vi "Set_All_Outputs.vi"(2 "error in":errorcluster, 3 "register 2 (8-13)":T1=[FALSE, FALSE, FALSE, FALSE, FALSE, FALSE], 4 "register 1 (2-7)":T2, 5 "VISA arduino in":refnum<visa-resource-name>) -> (0 "error out":errorcluster, 1 "VISA arduino out":refnum<visa-resource-name>)   [LabVIEW 2021]
uses:
  Register_1.ctl
  Register_2.ctl
  Delay_Global.vi
  <vilib>/Utility/error.llb/Error Cluster From Error Code.vi
  <vilib>/ErrorRing/Error Ring.xnode
panel:
  out "delay":u32
  out "comand 2":string
  out "comand 1":string
  # "Private"
  # "Public"
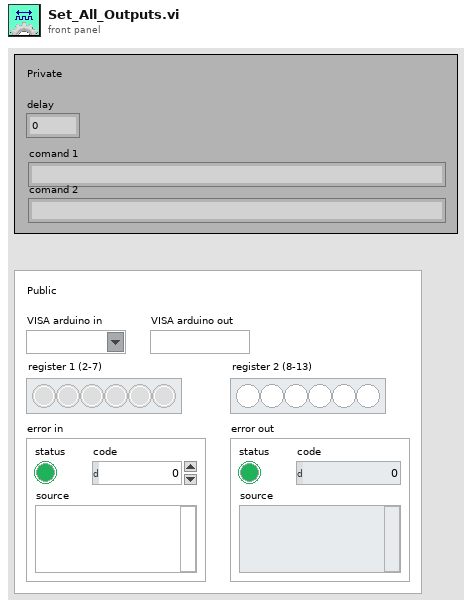
[diagram p1: front panel]
types:
  T1 = typedef "Register_2.ctl" = bool[]
  T2 = typedef "Register_1.ctl" = bool[]
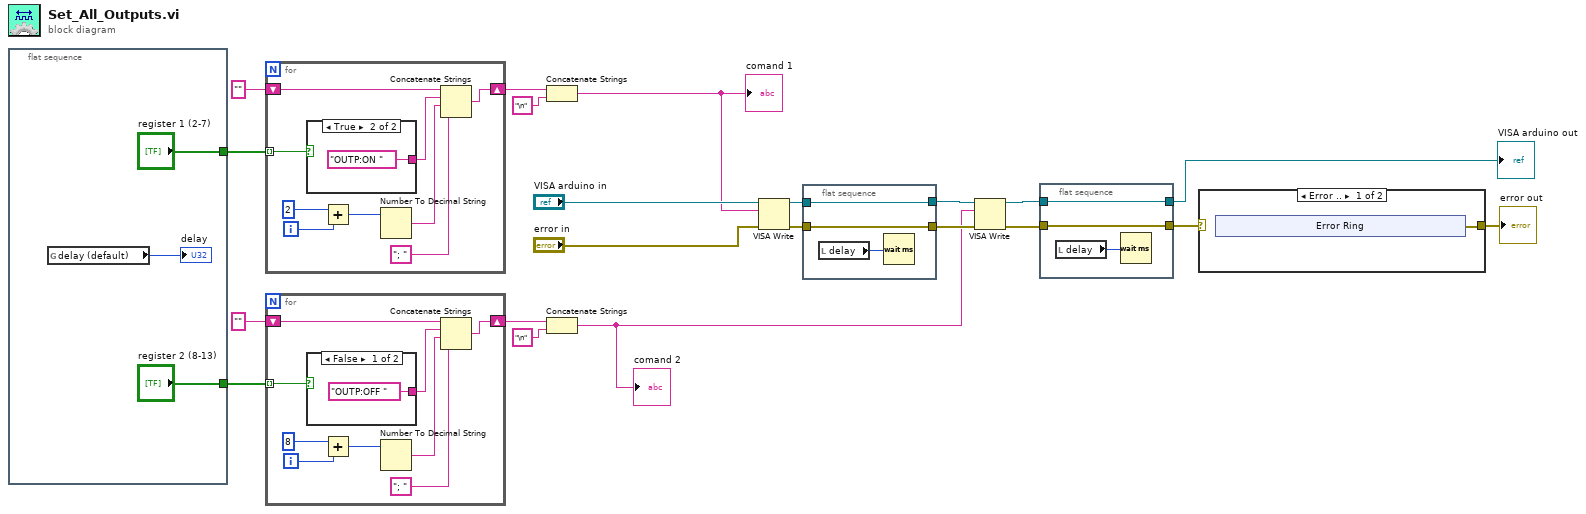
[diagram p0: block diagram]
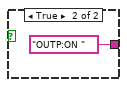
[diagram p3: hidden frame]
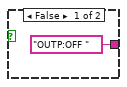
[diagram p4: hidden frame]
diagram:
  n1 = flat-sequence {
    tunnel: ["register 1 (2-7)"] -> w21
    tunnel: ["register 2 (8-13)"] -> w14
    frame #0 {
      n2 = global read "Delay_Global.vi" "delay (default)"() -> (→"delay":u32)
    }
  }
  n3 = for {
    shift-right: [w29] -> w18
    shift-left: "" -> [w28]
    tunnel: w21 -> [w33] mode=indexing
    i -> [w31]
    n4 = case shown="True" w33 {
      tunnel: ["OUTP:OFF " "OUTP:ON "] -> w27
      frame False {
      }
      frame True {
      }
    }
    n5 = Add(x=2, y=w31) -> (x+y=w30:i32)
    n6 = Number To Decimal String(number=w30) -> (decimal integer string=w26:string)  [unwired: 1 in]
    n7 = Concatenate Strings(w28, w27, w26, "; ") -> (w29:string)
  }
  n8 = for {
    shift-right: [w40] -> w17
    shift-left: "" -> [w39]
    tunnel: w14 -> [w44] mode=indexing
    i -> [w42]
    n9 = case shown="False" w44 {
      tunnel: ["OUTP:OFF " "OUTP:ON "] -> w38
      frame False {
      }
      frame True {
      }
    }
    n10 = Add(x=8, y=w42) -> (x+y=w41:i32)
    n11 = Number To Decimal String(number=w41) -> (decimal integer string=w37:string)  [unwired: 1 in]
    n12 = Concatenate Strings(w39, w38, w37, "; ") -> (w40:string)
  }
  n13 = Concatenate Strings(w18, "\n" ("string")) -> (w11:string)
  "comand 1" <- w11
  n14 = Concatenate Strings(w17, "\n" ("string")) -> (w6:string)
  "comand 2" <- w6
  n15 = VISA Write(VISA resource name="VISA arduino in", write buffer=w11, error in (no error)="error in") -> (VISA resource name out=w10:refnum<visa-resource-name>, error out=w9:errorcluster)  [unwired: 1 out]
  n16 = flat-sequence {
    tunnel: w10 -> [w48]
    tunnel: w9 -> [w47]
    tunnel: [w48] -> w8
    tunnel: [w47] -> w7
    frame #0 {
      n17 = local read "delay"() -> (w49:u32)
      n18 = Wait (ms)(milliseconds to wait=w49) -> ()  [unwired: 1 out]
    }
  }
  n19 = VISA Write(VISA resource name=w8, write buffer=w6, error in (no error)=w7) -> (VISA resource name out=w5:refnum<visa-resource-name>, error out=w4:errorcluster)  [unwired: 1 out]
  n20 = flat-sequence {
    tunnel: w5 -> [w50]
    tunnel: w4 -> [w51]
    tunnel: [w51] -> w3
    tunnel: [w50] -> w1
    frame #0 {
      n21 = local read "delay"() -> (w52:u32)
      n22 = Wait (ms)(milliseconds to wait=w52) -> ()  [unwired: 1 out]
    }
  }
  n23 = case shown="Error .." w3 {
    selector: w3 -> [_ w59]
    tunnel: [w53 w59] -> w2
    frame Error {
      n24 = xnode "Error Ring"() -> ("error out"=w53:errorcluster)
    }
    frame No Error {
    }
  }
  "error out" <- w2
  "VISA arduino out" <- w1
